vi "Read Diagnostic Values.vi"(7 "Unit Address (1)":u8=1, 8 "error in (no error)":errorcluster, 11 "VISA resource name":refnum<visa-resource-name>) -> (0 "error out":errorcluster, 1 "Loop Break Alarm":bool, 2 "Calculated Error":i32, 3 "VISA resource name out":refnum<visa-resource-name>, 4 "Sensor Break Status":bool)   [LabVIEW 2014, in "Eurotherm 35xx Series.lvlib"]
doc: "This VI returns Diagnostic Values."
uses:
  <instrlib>/Eurotherm 35xx Series/Eurotherm 35xx Series.lvlib
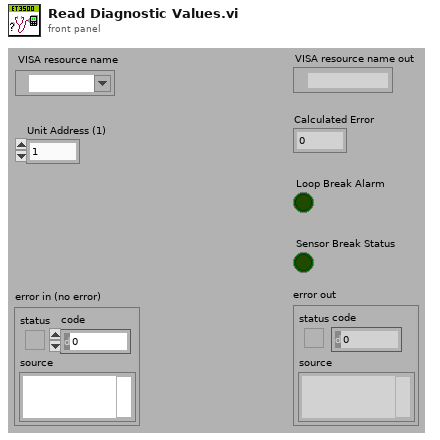
[diagram p1: front panel]
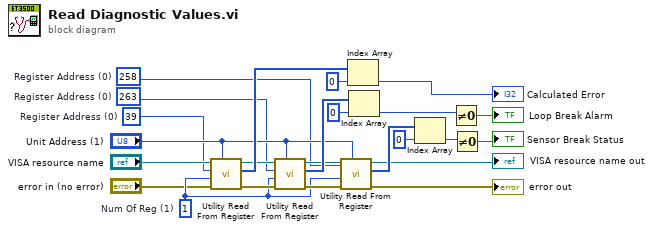
[diagram p0: block diagram]
diagram:
  w8 = 258  # Register Address (0)
  w7 = 263  # Register Address (0)
  w6 = 39  # Register Address (0)
  w14 = u16 1  # Num Of Reg (1)
  n1 = call <instrlib>:"Utility Read From Register.vi"("Unit Address (1)"="Unit Address (1)", "error in (no error)"="error in (no error)", "Num Of Reg (1)"=w14, "Register Address (0)"=w6, "VISA resource name"="VISA resource name") -> ("error out"=w15:errorcluster, "Data"=w24:i16[], "VISA resource name out"=w18:refnum<visa-resource-name>)  [unwired: 4 in]
  n2 = call <instrlib>:"Utility Read From Register.vi"("Unit Address (1)"="Unit Address (1)", "error in (no error)"=w15, "Num Of Reg (1)"=w14, "Register Address (0)"=w7, "VISA resource name"=w18) -> ("error out"=w16:errorcluster, "Data"=w21:i16[], "VISA resource name out"=w17:refnum<visa-resource-name>)  [unwired: 4 in]
  n3 = call <instrlib>:"Utility Read From Register.vi"("Unit Address (1)"="Unit Address (1)", "error in (no error)"=w16, "Num Of Reg (1)"=w14, "Register Address (0)"=w8, "VISA resource name"=w17) -> ("error out"=→"error out":errorcluster, "Data"=w20:i16[], "VISA resource name out"=→"VISA resource name out":refnum<visa-resource-name>)  [unwired: 4 in]
  n4 = Index Array(array=w24, index=0) -> (element=→"Calculated Error":i16)
  n5 = Index Array(array=w21, index=0) -> (element=w4:i16)
  n6 = Index Array(array=w20, index=0) -> (element=w2:i16)
  n7 = Not Equal To 0?(x=w4) -> (x != 0?=→"Loop Break Alarm":bool)
  n8 = Not Equal To 0?(x=w2) -> (x != 0?=→"Sensor Break Status":bool)
